vi "Hello World.vi"   [LabVIEW 2017]
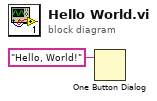
[diagram p0: block diagram]
diagram:
  n1 = One Button Dialog(message="Hello, World!" ("消息")) -> ()  [unwired: 1 in, 1 out]
